vi "pumpenable.vi"(7 "LabVIEW Web Service Request":refnum<class "Web Request.lvclass">) -> ()   [LabVIEW 2013]
uses:
  <vilib>/wsapi/Web Request.lvclass
  Controls/Test Action.ctl
panel:
  # "Use the Web Service Request input terminal to call the VIs on the Web Services palette. Do not remove it from the connector pane unless you don't need access to the palette."
  # "Each additional control wired to the connector pane will be available as an input in the URL. To include an indicator in terminal-mode output (the default setting), it must also be wired to the connector pane."
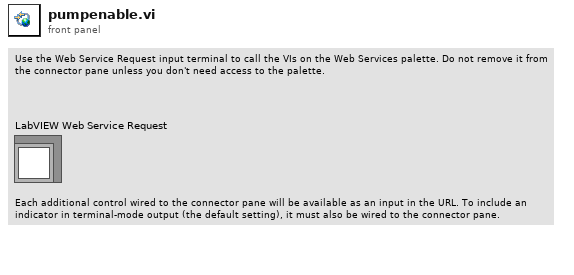
[diagram p1: front panel]
types:
  T1 = typedef "Test Action.ctl" = enum16{"Idle", "Start", "Stop", "Pump Cmd", "Pump 1 Enable", "Pump 2 Enable", "Pump 3 Enable", "Pump 4 Enable", "Pump 5 Enable", "Pump 6 Enable", "Timer 1 Reset", "Timer 2 Reset", "Timer 3 Reset", "Timer 4 Reset", "Timer 5 Reset", "Timer 6 Reset"}
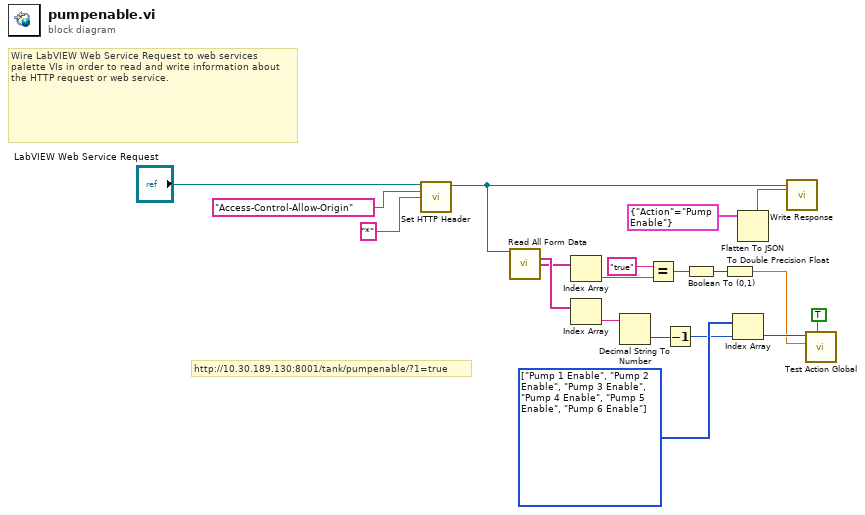
[diagram p0: block diagram]
diagram:
  w9 = T1[] [enum."Pump 1 Enable", enum."Pump 2 Enable", enum."Pump 3 Enable", enum."Pump 4 Enable", enum."Pump 5 Enable", enum."Pump 6 Enable"] items=["Idle", "Start", "Stop", "Pump Cmd", "Pump 1 Enable", "Pump 2 Enable", "Pump 3 Enable", "Pump 4 Enable", "Pump 5 Enable", "Pump 6 Enable", "Timer 1 Reset", "Timer 2 Reset", "Timer 3 Reset", "Timer 4 Reset", "Timer 5 Reset", "Timer 6 Reset"]
  # "http://10.30.189.130:8001/tank/pumpenable/?1=true"
  # "Wire LabVIEW Web Service Request to web services palette VIs in order to read and write information about the HTTP request or web service."
  n1 = call <vilib>:"Set HTTP Header.vi"("LabVIEW Web Service Request"="LabVIEW Web Service Request", "header"="Access-Control-Allow-Origin" ("header value"), "header value"="*" ("header")) -> ("LabVIEW Web Service Request out"=w13:refnum<class "Web Request.lvclass">)  [unwired: 11 in, 1 out]
  n2 = call <vilib>:"Read All Form Data.vi"("LabVIEW Web Service Request"=w13) -> ("Key"=w12:string[], "Value"=w6:string[])  [unwired: 10 in, 3 out]
  n3 = Index Array(array=w6) -> (element=w5:string)  [unwired: 1 in]
  n4 = Index Array(array=w12) -> (element=w11:string)  [unwired: 1 in]
  n5 = Decimal String To Number(string=w11) -> (number=w10:i32)  [unwired: 2 in, 1 out]
  n6 = Equal?(x="true", y=w5) -> (x = y?=w3:bool)
  n7 = Decrement(x=w10) -> (x-1=w8:i32)
  n8 = Boolean To (0,1)(Boolean=w3) -> (0, 1=w2:i16)
  n9 = To Double Precision Float(number=w2) -> (double precision float=w1:dbl)
  n10 = Index Array(array=w9, index=w8) -> (element=w7:T1)
  n11 = Flatten To JSON(anything=cluster{"Action":string} {"Action"="Pump Enable"}) -> (JSON string=w16:string)  [unwired: 2 in, 1 out]
  n12 = call <vilib>:"Write Response.vi"("LabVIEW Web Service Request"=w13, "response string"=w16) -> ()  [unwired: 12 in, 2 out]
  n13 = call "Test Action Global.vi"("Write (F)"=TRUE, "Data IN"=w1, "Test Action IN"=w7) -> ()  [unwired: 7 in, 2 out]
